vi "Event Handle Loop_Pop-out Panel.vi"(8 "error in (no error)":errorcluster, 11 "QTab Class in":refnum<class "QTab Class.lvclass">) -> (0 "error out":errorcluster)   [LabVIEW 2020, in "QTab.lvlib" / "QTab Class.lvclass"]
uses:
  QTab Class.lvclass
  QTab Class.lvclass/QTab Class.ctl
  Pag Attribute.ctl
  Command.ctl
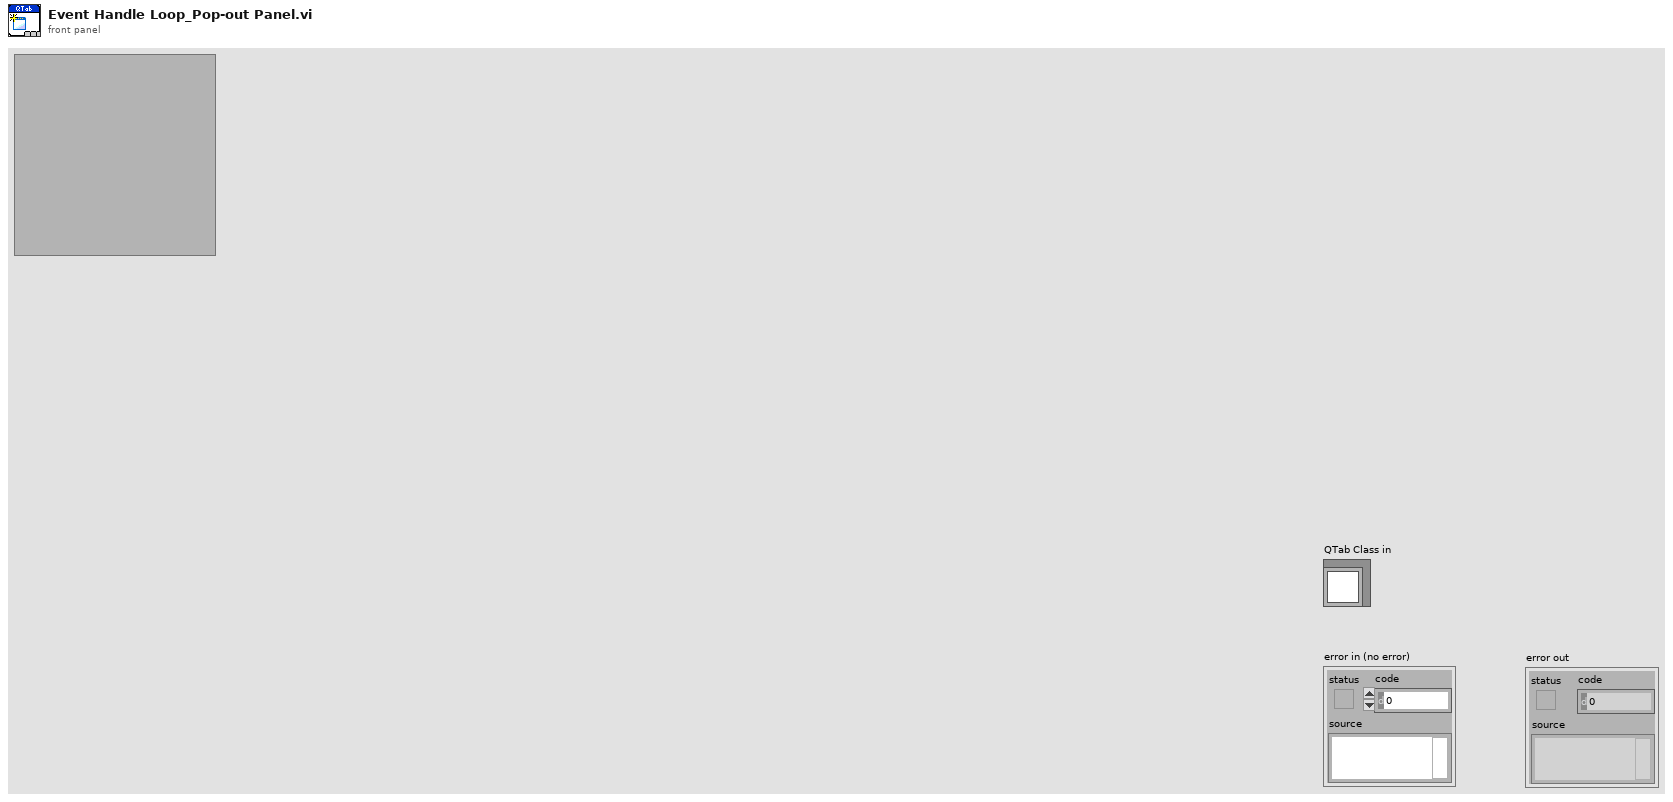
[diagram p1: front panel]
types:
  T1 = typedef "QTab.lvlib/QTab Class.lvclass/Pag Attribute.ctl" = cluster{"VI Refnum":refnum<vi>, "Page Name":string, "Closeable":bool, "Draggable":bool, "Pop-Out":bool}
  T2 = enum32{"Invalid", "Standard", "Closed", "Hidden", "Minimized", "Maximized"}
  T3 = typedef "QTab.lvlib/QTab Class.lvclass/Command.ctl" = enum16{"Startup", "Add Page", "Close All Page", "Set Page Attribute", "Pop-out", "Merage", "Insert", "Stop"}
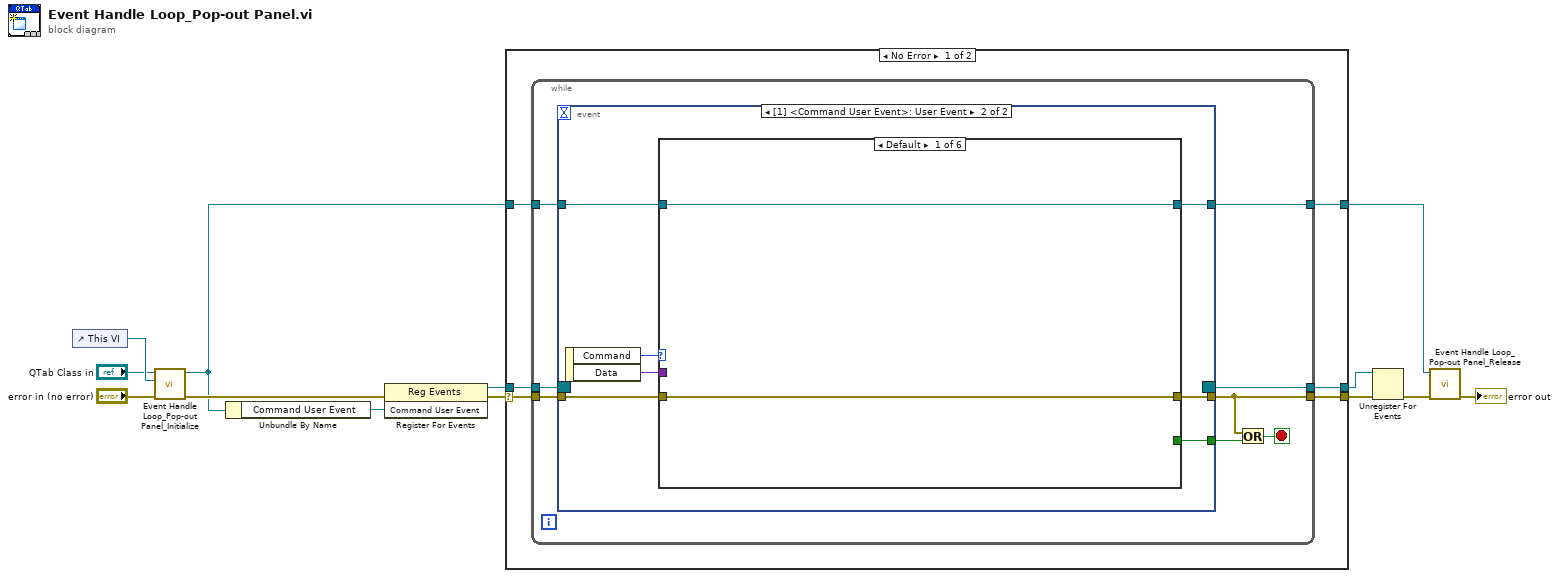
[diagram p0: block diagram]
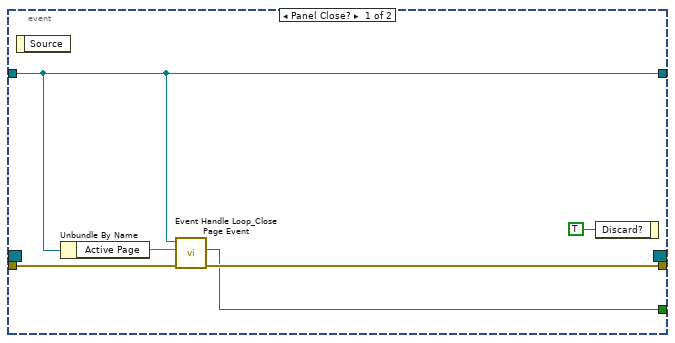
[diagram p2: hidden frame]
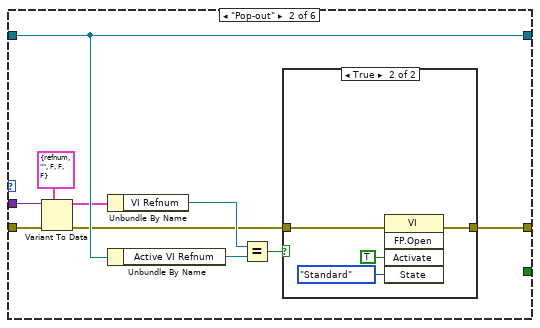
[diagram p3: hidden frame]
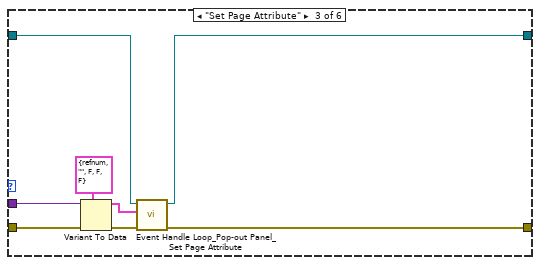
[diagram p5: hidden frame]
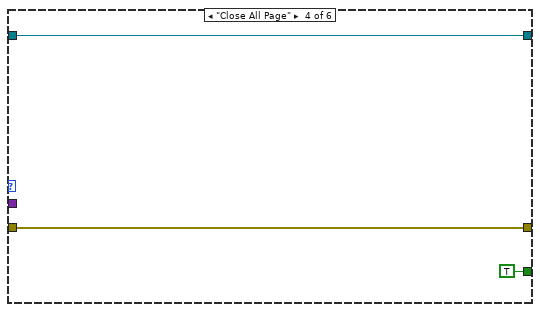
[diagram p6: hidden frame]
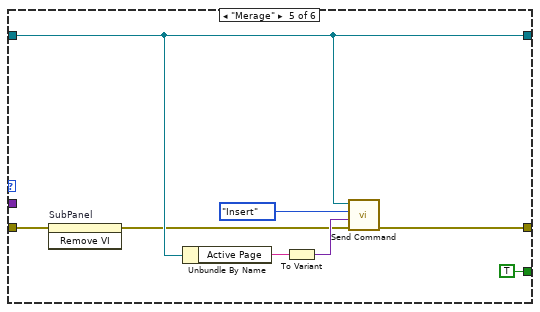
[diagram p7: hidden frame]
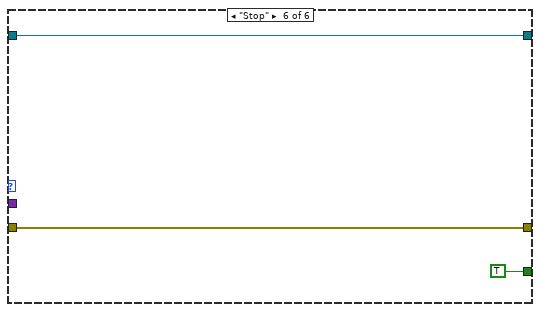
[diagram p8: hidden frame]
diagram:
  n1 = control-ref of="This VI"() -> (w7:refnum<vi>)
  n2 = call "Event Handle Loop_Pop-out Panel_Initialize.vi"("error in (no error)"="error in (no error)", "VI Refnum"=w7, "QTab Class in"="QTab Class in") -> ("error out"=w5:errorcluster, "QTab Class out"=w4:refnum<class "QTab Class.lvclass">)  [unwired: 7 in]
  n3 = Unbundle By Name(w4) -> ("Command User Event"=w13:refnum<user-event>)
  n4 = register-events(error in=w5, w13) -> (reference out=w11:refnum<event-registration>, error out=w12:errorcluster)  [unwired: 1 in]
  n5 = case shown="No Error" w12 {
    selector: w12 -> [w18 w81]
    tunnel: w4 -> [w19 w82]
    tunnel: w11 -> [w17 w80]
    tunnel: [w16 w82] -> w2
    tunnel: [w15 w81] -> w10
    tunnel: [w14 w80] -> w9
    frame No Error {
      n6 = while {
        tunnel: w19 -> [w26]
        tunnel: w18 -> [w27]
        tunnel: w17 -> [w25]
        tunnel: [w24] -> w16
        tunnel: [w22] -> w15
        tunnel: [w20] -> w14
        stop <- w21 stop-if-true
        n7 = event shown="[1] <Command User Event>: User Event" {
          selector: w25 -> [_ _]
          dyn-events: [_ _] -> w20
          timeout: _ -> [_ _]
          tunnel: w27 -> [w32 w38]
          tunnel: w26 -> [w30 w39]
          tunnel: [w30 w35] -> w24
          tunnel: [w29 w37] -> w22
          tunnel: [w28 w36] -> w23
          event Panel Close? {
            n8 = event-data() -> ()  [unwired: 1 in, 1 out]
            n9 = Unbundle By Name(w30) -> ("Active Page"=w31:string)
            n10 = call "Event Handle Loop_Close Page Event.vi"("error in (no error)"=w32, "Label"=w31, "QTab Class in"=w30) -> ("error out"=w29:errorcluster, "Confirm"=w28:bool)  [unwired: 6 in, 1 out]
            n11 = event-data("Discard?"=TRUE) -> ()  [unwired: 1 in, 1 out]
          }
          event User Event {
            n12 = event-data() -> ("Command"=w34:T3, "Data"=w40:variant)  [unwired: 1 in]
            n13 = case shown="Default" w34 {
              tunnel: w40 -> [_ w51 w64 _ _ _]
              tunnel: w39 -> [w42 w49 w61 w68 w74 w79]
              tunnel: [w42 w49 w59 w68 w74 w79] -> w35
              tunnel: w38 -> [w41 w52 w65 w67 w71 w78]
              tunnel: [w41 w43 w58 w67 w76 w78] -> w37
              tunnel: [_ _ _ TRUE TRUE TRUE] -> w36
              frame Default {
              }
              frame "Pop-out" {
                n14 = Variant To Data(error in=w52, type=T1 {"VI Refnum"=refnum, "Page Name"="", "Closeable"=FALSE, "Draggable"=FALSE, "Pop-Out"=FALSE} ("Pag Attribute"), Variant=w51) -> (data=w48:T1, error out=w44:errorcluster)
                n15 = Unbundle By Name(w48) -> ("VI Refnum"=w46:refnum<vi>)
                n16 = Unbundle By Name(w49) -> ("Active VI Refnum"=w47:refnum<vi>)
                n17 = Equal?(x=w46, y=w47) -> (x = y?=w45:bool)
                n18 = case shown="True" w45 {
                  tunnel: w44 -> [w53 w57]
                  tunnel: [w53 w56] -> w43
                  frame False {
                  }
                  frame True {
                    n19 = invoke class="VI" method="FP.Open"(error in=w57, "Activate"=TRUE ("Activate?"), "State"=T2."Standard") -> (error out=w56:errorcluster)  [unwired: 2 in, 4 out]
                  }
                }
              }
              frame "Set Page Attribute" {
                n20 = Variant To Data(error in=w65, type=T1 {"VI Refnum"=refnum, "Page Name"="", "Closeable"=FALSE, "Draggable"=FALSE, "Pop-Out"=FALSE} ("Pag Attribute"), Variant=w64) -> (data=w60:T1, error out=w62:errorcluster)
                n21 = call "Event Handle Loop_Pop-out Panel_Set Page Attribute.vi"("error in (no error)"=w62, "Pag Attribute"=w60, "QTab Class in"=w61) -> ("error out"=w58:errorcluster, "QTab Class out"=w59:refnum<class "QTab Class.lvclass">)  [unwired: 7 in]
              }
              frame "Close All Page" {
              }
              frame "Merage" {
                n22 = invoke on="SubPanel" class="SubPnl" method="Remove VI"(error in=w71) -> (error out=w70:errorcluster)  [unwired: 2 in, 2 out]
                n23 = Unbundle By Name(w74) -> ("Active Page"=w73:string)
                n24 = To Variant(anything=w73) -> (Variant=w72:variant)
                n25 = call "Send Command.vi"("error in (no error)"=w70, "Data"=w72, "Command"=Command."Insert", "QTab Class in"=w74) -> ("error out"=w76:errorcluster)  [unwired: 6 in, 1 out]
              }
              frame "Stop" {
              }
            }
          }
        }
        n26 = Or(x=w22, y=w23) -> (x .or. y?=w21:bool)
      }
    }
    frame Error {
    }
  }
  n27 = Unregister For Events(event registration refnum=w9, error in=w10) -> (error out=w3:errorcluster)
  n28 = call "Event Handle Loop_Pop-out Panel_Release.vi"("error in (no error)"=w3, "QTab Class in"=w2) -> ("error out"=→"error out":errorcluster)  [unwired: 9 in]
